vi "StudentScope - Help.vi"() -> ()   [LabVIEW 2015]
panel:
  out "String":string="Introduction\n\nThe StudentScope is a software oscilloscope specifically designed to work with the National Instruments USB-6009 data acquisition device. To simulate the functionality of a scope, the StudentScope acquires analog input data across two channels and then searches for a user-specified trigger level. This allows periodic waveforms to be lined up and displayed as standing waves. Controls to scale signals, apply vertical offsets, adjust the timebase, and measure phase offsets are all meant to function similarly to a benchtop oscilloscope. Several expanded features are also available, including a option to log data to an Excel-compatible spreadsheet file or to export a screenshot to a printable HTML report.\n\nGetting Started\n\nFirst, be sure you have the LabVIEW Run-Time Engine version 8.0 and the DAQmx driver version 8.0 or later installed under the default installation options. Both can be downloaded free of charge from ni.com. Next, connect your National Instruments USB-6009 to your PC. Windows should detect the device and configure the appropriate driver. If this is the first time that a USB-6009 device is installed on your computer, you might be prompted to install a USB-6xxx Firmware Loader. Please complete the Windows Hardware Wizard prompts to completely install this device.\n\nTo run the StudentScope, you will need to determine the device number of your USB-6009, which is how the hardware is identified by the scope software. Find this by opening National Instruments Measurement and Automation Explorer (MAX). In MAX, expand Devices and Interfaces. Then expand NI-DAQmx Devices. If the DAQmx driver is installed properly, and the USB-6009 is connected, you will see an item such as USB-6009: \"Dev1\" where Dev1 indicates device # 1. Make a note of the device number.\n\nWhen you run the StudentScope, you will need to select the correct device number. If the wrong device number is selected, you will receive an error message. To fix this, be sure the USB-6009 plugged in, select the correct device number, and press the reset button. \n\nHardware Connections\n\nConnect input signals to differential channels 0 and 1 on the USB-6009. Terminals 2 and 3 on the 6009 correspond to the positive and negative inputs for differential channel 0. Terminals 5 and 6 the 6009 correspond to the positive and negative inputs for differential channel 1. For more information on terminals and connections, consult the help manual for the device.\n\nControls\n\nDevice: Specifies the Device Number of the 6009, which uniquely identifies the hardware. This number can be found in Measurement and Automation Explorer (MAX). If you adjust this input, you will have to press reset for the changes to take effect.\n\nChannels: Specifies the number of channels to scan. By acquiring only a single channel of data, twice the sampling rate can be achieved over acquiring two channels of data. If you adjust this input, you will have to press reset for the changes to take effect.\n\nInput Voltage Range: Sets the internal programmable gain amplifier on the 6009. This applies an appropriate analog gain to the signal prior to digitization. For best results, choose the smallest range setting that completely encapsulates the expected signal. If you adjust this input, you will have to press reset for the changes to take effect.\n\nReset: If Device, Channels, or Input Voltage Range values are changed, the StudentScope needs to be reset for the changes to take effect.\n\nDisplay On: Toggles the visibility of each channel's trace. Note: This does not change whether or not the data is actually being acquired by the USB-6009; it merely allows the user to turn on or off the display of that data.\n\nOffset: Adjusts the vertical position of the trace on the display by adding or subtracting a voltage offset.\n\nZero: Removes any offsets added with the Offset knob.\n\nCenter:  Automatically adjusts the Offset knob so that the waveform is centered vertically on the display.\n\nScale: Sets the Volts per division along the vertical axis in order to \"zoom\" vertically.\n\nTimebase: Sets the time per division along the horizontal axis in order to \"zoom\" horizontally. This does not change the rate of acquisition of the hardware.\n\nTrigger Channel: Specifies which channel will generate the trigger.\n\nEdge: Toggles between triggering off of a rising or falling edge of the signal.\n \nLevel: Specifies the voltage level at which a trigger will be generated. Note: If the level is never crossed by the periodic signal, the trigger will not work properly and the waveform will not display correctly. Also, the trigger is defined in software, and will only correctly display periodic signals with a period of less than 1/8 second.  \n\nCursors (On/Off): Toggles display of the cursors on or off. \n\nLock Cursors: Toggles whether cursors are free-floating or locked to a channel trace. If cursors are free floating, the voltage level at each cursor will not be displayed. \n\nC1: If Lock Cursors is toggle on, this selects the channel to which Cursor 1 is locked.\n\nC2: If Lock Cursors is toggle on, this selects the channel to which Cursor 2 is locked.\n"
  in  "Help":bool
  # "StudentScope for USB 6009"
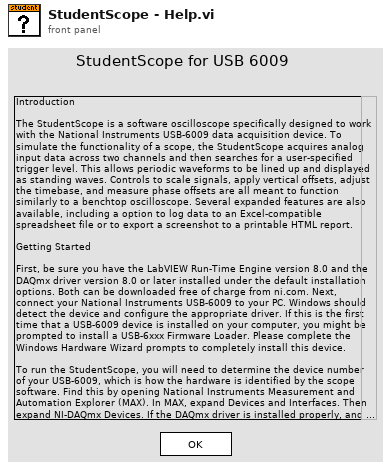
[diagram p1: front panel]
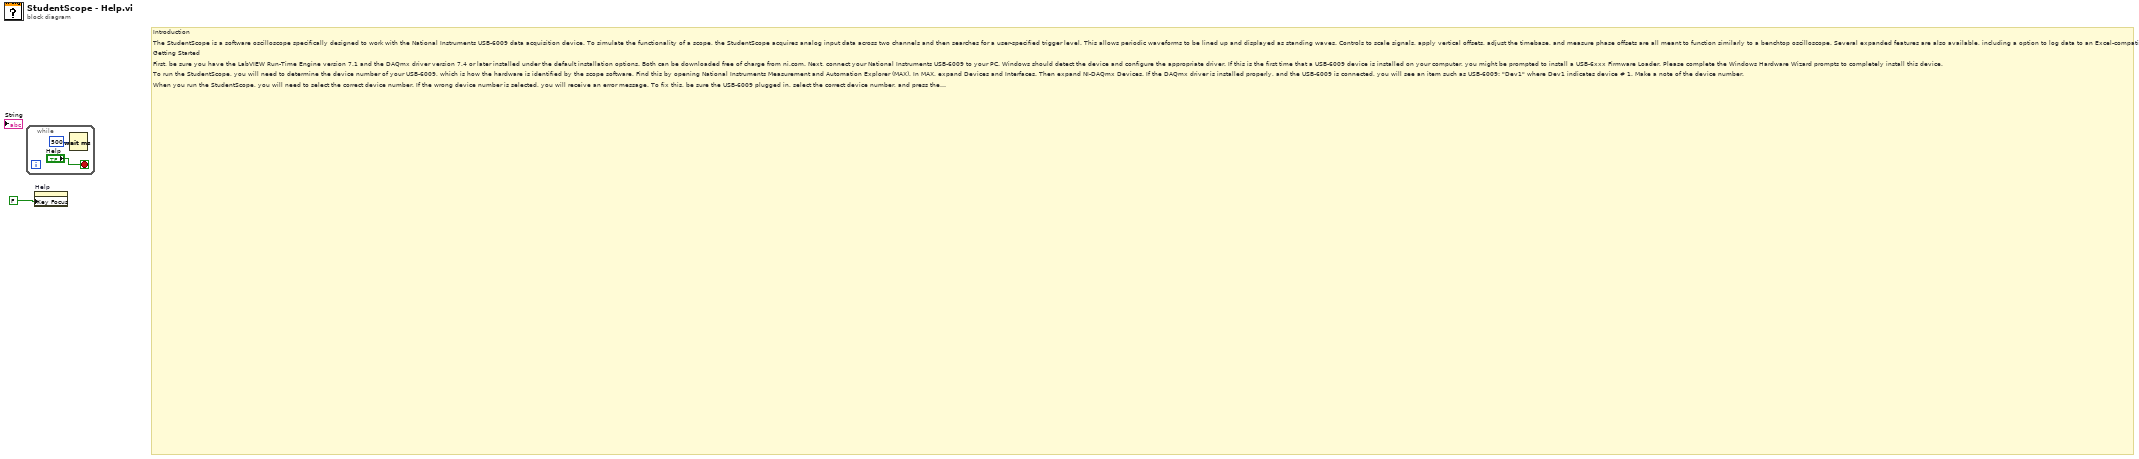
[diagram p0: block diagram]
diagram:
  # "Introduction\n\nThe StudentScope is a software oscilloscope specifically designed to work with the National Instruments USB-6009 data acquisition device. To simulate the functionality of a scope, the StudentScope acquires analog input data across two channels and then searches for a user-specified trigger level. This allows periodic waveforms to be lined up and displayed as standing waves. Controls to scale signals, apply vertical offsets, adjust the timebase, and measure phase offsets are all meant to function similarly to a benchtop oscilloscope. Several expanded features are also available, including a option to log data to an Excel-compatible spreadsheet file.\n\nGetting Started\n\nFirst, be sure you have the LabVIEW Run-Time Engine version 7.1 and the DAQmx driver version 7.4 or later installed under the default installation options. Both can be downloaded free of charge from ni.com. Next, connect your National Instruments USB-6009 to your PC. Windows should detect the device and configure the appropriate driver. If this is the first time that a USB-6009 device is installed on your computer, you might be prompted to install a USB-6xxx Firmware Loader. Please complete the Windows Hardware Wizard prompts to completely install this device.\n\nTo run the StudentScope, you will need to determine the device number of your USB-6009, which is how the hardware is identified by the scope software. Find this by opening National Instruments Measurement and Automation Explorer (MAX). In MAX, expand Devices and Interfaces. Then expand NI-DAQmx Devices. If the DAQmx driver is installed properly, and the USB-6009 is connected, you will see an item such as USB-6009: \"Dev1\" where Dev1 indicates device # 1. Make a note of the device number.\n\nWhen you run the StudentScope, you will need to select the correct device number. If the wrong device number is selected, you will receive an error message. To fix this, be sure the USB-6009 plugged in, select the correct device number, and press the reset button. \n\nHardware Connections\n\nConnect input signals to differential channels 0 and 1 on the USB-6009. Terminals 2 and 3 on the 6009 correspond to the positive and negative inputs for differential channel 0. Terminals 5 and 6 the 6009 correspond to the positive and negative inputs for differential channel 1. For more information on terminals and connections, consult the help manual for the device.\n\nControls\n\nDevice: Specifies the Device Number of the 6009, which uniquely identifies the hardware. This number can be found in Measurement and Automation Explorer (MAX). If you adjust this input, you will have to press reset for the changes to take effect.\n\nChannels: Specifies the number of channels to scan. By acquiring only a single channel of data, twice the sampling rate can be achieved over acquiring two channels of data. If you adjust this input, you will have to press reset for the changes to take effect.\n\nInput Voltage Range: Sets the internal programmable gain amplifier on the 6009. This applies an appropriate analog gain to the signal prior to digitization. For best results, choose the smallest range setting that completely encapsulates the expected signal. If you adjust this input, you will have to press reset for the changes to take effect.\n\nReset: If Device, Channels, or Input Voltage Range values are changed, the StudentScope needs to be reset for the changes to take effect.\n\nDisplay On: Toggles the visibility of each channel's trace. Note: This does not change whether or not the data is actually being acquired by the USB-6009; it merely allows the user to turn on or off the display of that data.\n\nOffset: Adjusts the vertical position of the trace on the display by adding or subtracting a voltage offset.\n\nZero: Removes any offsets added with the Offset knob.\n\nScale: Sets the Volts per division along the vertical axis in order to \"zoom\" vertically.\n\nTimebase: Sets the time per division along the horizontal axis in order to \"zoom\" horizontally. This does not change the rate of acquisition of the hardware.\n\nTrigger Channel: Specifies which channel will generate the trigger.\n\nEdge: Toggles between triggering off of a rising or falling edge of the signal.\n \nLevel: Specifies the voltage level at which a trigger will be generated. Note: If the level is never crossed by the periodic signal, the trigger will not work properly and the waveform will not display correctly.\n\nCursors (On/Off): Toggles display of the cursors on or off. \n\nLock Cursors: Toggles whether cursors are free-floating or locked to a channel trace. If cursors are free floating, the voltage level at each cursor will not be displayed. \n\nC1: If Lock Cursors is toggle on, this selects the channel to which Cursor 1 is locked.\n\nC2: If Lock Cursors is toggle on, this selects the channel to which Cursor 2 is locked."
  n1 = while {
    stop <- "Help" stop-if-true
    n2 = Wait (ms)(milliseconds to wait=u32 500) -> ()  [unwired: 1 out]
  }
  n3 = property on="Help" class="Bool"("Key Focus"=FALSE) -> ()  [unwired: 2 in, 2 out]
